vi "deinitialize.vi"(0 "HB_Simple":refnum<class "HB_Simple.lvclass">, 5 "error in (no error)":errorcluster) -> (19 "error out":errorcluster)   [LabVIEW 2009, in "HB_BaseClass_Examples.lvlib" / "HB_Simple.lvclass"]
doc: "This is a dynamic dispatch VI. It can be overwritten by childclasses to release allocated recources."
uses:
  HB_Simple.lvclass
  lib.lib/HGF_LVC/HGF_BaseClasses/HGF_Visitable/HGF_Visitable.lvclass
  HB_Simple.lvclass/HB_Simple.ctl
  lib.lib/HGF_LVC/HGF_BaseClasses/HGF_Factory/HGF_Factory.lvclass
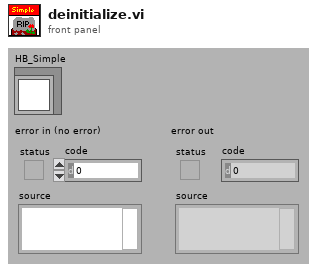
[diagram p1: front panel]
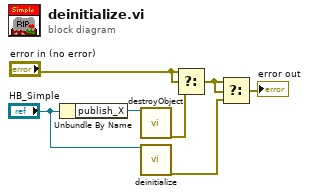
[diagram p0: block diagram]
diagram:
  n1 = Unbundle By Name("HB_Simple") -> ("publish_X"=w2:refnum<class "HGF_PVPublisher.lvclass">)
  n2 = call "destroyObject.vi"("HGF_Factory"=w2) -> ("error out"=w1:errorcluster)  [unwired: 18 in]
  n3 = call-parent "deinitialize.vi"("HGF_Factory"="HB_Simple") -> ("error out"=w4:errorcluster)  [unwired: 1 in, 17 out]
  n4 = Select(t="error in (no error)", s="error in (no error)", f=w1) -> (s? t:f=w5:errorcluster)
  n5 = Select(t=w5, s=w5, f=w4) -> (s? t:f=→"error out":errorcluster)
